vi "reference_maker2.vi"(8 "Raw_PPG":dbl[](array[numeric]), 11 "start_index":i32) -> (3 "reference":dbl[](array[numeric]))   [LabVIEW 2014]
panel:
  out "size":dbl
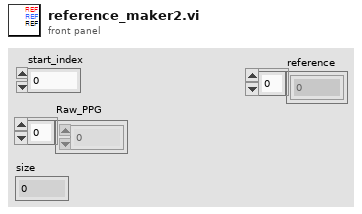
[diagram p1: front panel]
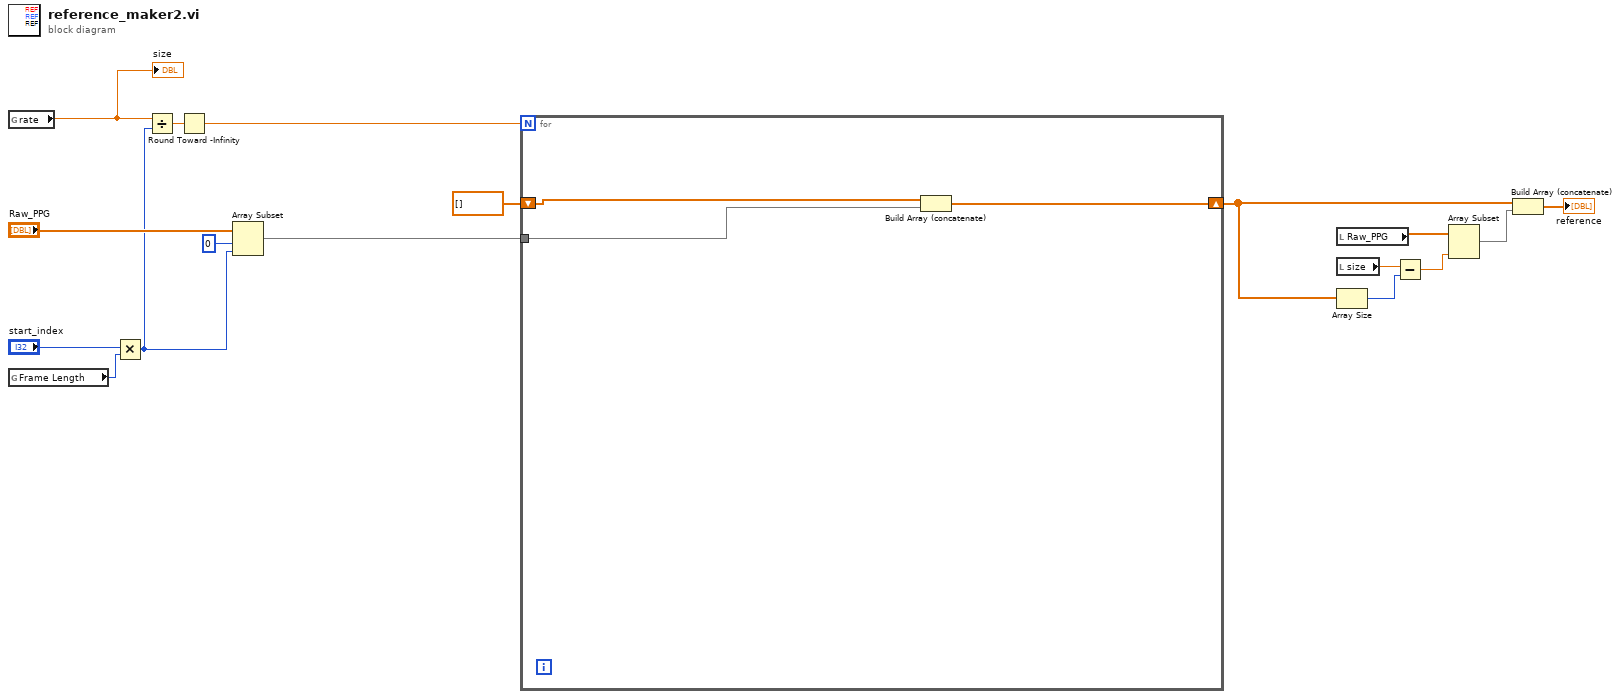
[diagram p0: block diagram]
diagram:
  n1 = global read "Control_Panel.vi" "rate"() -> (w1:dbl)
  "size" <- w1
  n2 = global read "Control_Panel.vi" "Frame Length"() -> (w16:i32)
  n3 = Multiply(x="start_index", y=w16) -> (x*y=w13:i32)
  n4 = Divide(x=w1, y=w13) -> (x/y=w12:dbl)
  n5 = Round Toward -Infinity(1:w12) -> (0:w9:dbl)
  n6 = Array Subset(array="Raw_PPG", index=0, length=w13) -> (w11:dbl[])
  n7 = for {
    N: w9 -> [_]
    tunnel: w11 -> [w20]
    shift-right: [w19] -> w4
    shift-left: dbl[] [] -> [w18]
    n8 = Build Array (concatenate)(w18, w20) -> (w19:dbl[])
  }
  n9 = local read "Raw_PPG"() -> (w5:dbl[])
  n10 = local read "size"() -> (w8:dbl)
  n11 = Array Size(array=w4) -> (size(s)=w7:i32)
  n12 = Subtract(x=w8, y=w7) -> (x-y=w6:dbl)
  n13 = Array Subset(array=w5, length=w6) -> (w3:dbl[])  [unwired: 1 in]
  n14 = Build Array (concatenate)(w4, w3) -> (→"reference":dbl[])
